vi "SVT STFT vs Time.vi"   [LabVIEW 2017, in "SoundVib_Transient.lvlib"]
doc: "Performs a short-time Fourier transform (STFT) on <B>scaled signal [EU]</B> and returns the power spectrum, waterfall, or colormap at the various times you specify. Wire data to the <B>scaled signal [EU]</B> input to determine the polymorphic instance to use or manually select the instance."
uses:
  <vilib>/addons/Sound and Vibration/svt_Transients/SoundVib_Transient.lvlib
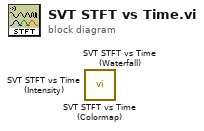
[diagram p0: block diagram]
diagram:
  n1 = call <vilib>:"SVT STFT vs Time (Colormap).vi"() -> ()  [unwired: 12 in, 4 out]
  n2 = call <vilib>:"SVT STFT vs Time (Waterfall).vi"() -> ()  [unwired: 12 in, 4 out]
  n3 = call <vilib>:"SVT STFT vs Time (Intensity).vi"() -> ()  [unwired: 10 in, 6 out]
